vi "Close all lasers.vi"(8 "error in":errorcluster, 11 "Laser cluster":T1) -> (0 "error out":errorcluster)   [LabVIEW 2017]
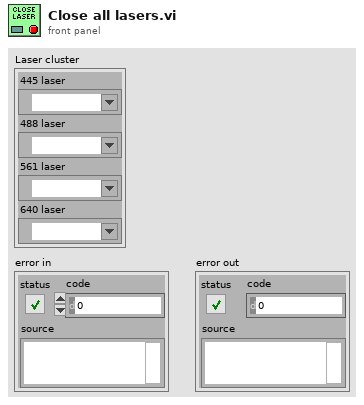
[diagram p1: front panel]
types:
  T1 = cluster{"445 laser":refnum<visa-resource-name>, "488 laser":refnum<visa-resource-name>, "561 laser":refnum<visa-resource-name>, "640 laser":refnum<visa-resource-name>}
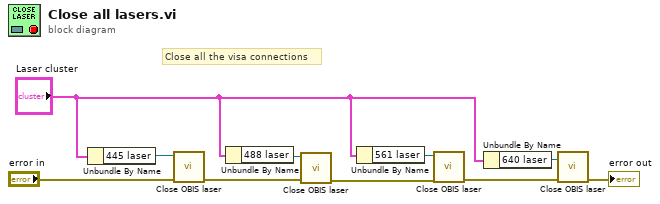
[diagram p0: block diagram]
diagram:
  # "Close all the visa connections"
  n1 = Unbundle By Name("Laser cluster") -> ("445 laser"=w5:refnum<visa-resource-name>)
  n2 = call "Close OBIS laser.vi"("error in"="error in", "VISA resource name"=w5) -> ("error out"=w9:errorcluster)  [unwired: 9 in]
  n3 = Unbundle By Name("Laser cluster") -> ("488 laser"=w2:refnum<visa-resource-name>)
  n4 = call "Close OBIS laser.vi"("error in"=w9, "VISA resource name"=w2) -> ("error out"=w8:errorcluster)  [unwired: 9 in]
  n5 = Unbundle By Name("Laser cluster") -> ("561 laser"=w3:refnum<visa-resource-name>)
  n6 = call "Close OBIS laser.vi"("error in"=w8, "VISA resource name"=w3) -> ("error out"=w7:errorcluster)  [unwired: 9 in]
  n7 = Unbundle By Name("Laser cluster") -> ("640 laser"=w4:refnum<visa-resource-name>)
  n8 = call "Close OBIS laser.vi"("error in"=w7, "VISA resource name"=w4) -> ("error out"=→"error out":errorcluster)  [unwired: 9 in]
